vi "DAC_2.vi"   [LabVIEW 2015]
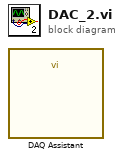
[diagram p0: block diagram]
diagram:
  n1 = call "DAQ Assistant"() -> ()  [unwired: 18 in, 2 out]
